vi "Convert Shutdown Furnace to Heater State Enum.vi"(10 "Shutdown Furnace?":bool) -> (2 "Heater State":T1)   [LabVIEW 2015, in "Thermal Chamber Controller_DQMH.lvlib"]
doc: "This VI converts the Furnace On/Off boolean to the Heater State enumerator.\n____\nDelacor QMH Thermal Chamber Examples 4.0.0.21\nCopyright (c) 2018, Delacor"
uses:
  Thermal Chamber Controller_DQMH.lvlib
  Heater State--enum.ctl
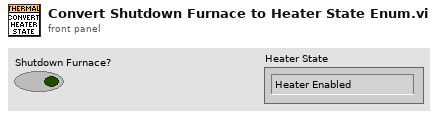
[diagram p1: front panel]
types:
  T1 = typedef "Thermal Chamber Controller_DQMH.lvlib/Heater State--enum.ctl" = enum16{"Heater Enabled", "Heater Disabled"}
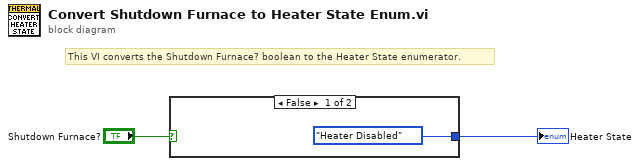
[diagram p0: block diagram]
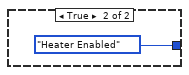
[diagram p2: hidden frame]
diagram:
  # "This VI converts the Shutdown Furnace? boolean to the Heater State enumerator."
  n1 = case shown="False" "Shutdown Furnace?" {
    tunnel: [Heater_State--enum."Heater Disabled" ("Heater State") Heater_State--enum."Heater Enabled" ("Heater State")] -> w1
    frame False {
    }
    frame True {
    }
  }
  "Heater State" <- w1
